vi "AddTestMethod_Item_CanDropItem.vi"(10 "DropItem":T1, 11 "Object":T1) -> (3 "CanDrop":bool)   [LabVIEW 2013]
uses:
  <resource>/Framework/Providers/API/ItemRef.ctl
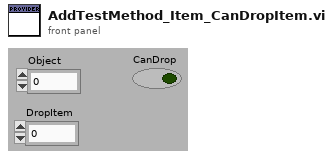
[diagram p1: front panel]
types:
  T1 = typedef "ItemRef.ctl" = u64
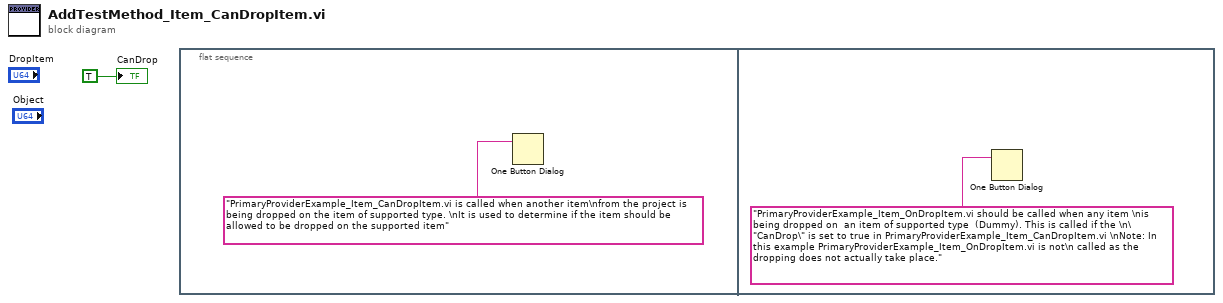
[diagram p0: block diagram]
diagram:
  n1 = flat-sequence {
    frame #0 {
      n2 = One Button Dialog(message="PrimaryProviderExample_Item_CanDropItem.vi is called when another item\nfrom the project is being dropped on the item of supported type. \nIt is used to determine if the item should be allowed to be dropped on the supported item") -> ()  [unwired: 1 in, 1 out]
    }
    frame #1 {
      n3 = One Button Dialog(message="PrimaryProviderExample_Item_OnDropItem.vi should be called when any item \nis being dropped on  an item of supported type  (Dummy). This is called if the \n\"CanDrop\" is set to true in PrimaryProviderExample_Item_CanDropItem.vi \nNote: In this example PrimaryProviderExample_Item_OnDropItem.vi is not\n called as the dropping does not actually take place." ("button name (\"OK\")")) -> ()  [unwired: 1 in, 1 out]
    }
  }
  "CanDrop" <- TRUE ("CanDrag")
